vi "ParseXML.vi"(8 "error in (no error)":errorcluster, 11 "Node":string="<Sequential ID=\"1\">\n<Parallel ID=\"2\">\n<Wait ID=\"6\" Time=\"1.00\"/>\n<DriveForDistance Distance=\"4.00\" ID=\"3\" Speed=\"4.00\"/>\n</Parallel>\n<DrivePath ID=\"5\" Path=\"2C\"/>\n</Sequential>\n</Sequential>") -> (0 "error out":errorcluster)   [LabVIEW 2017]
uses:
  <vilib>/regexp/Match Regular Expression.xnode
panel:
  out "Node Name":string
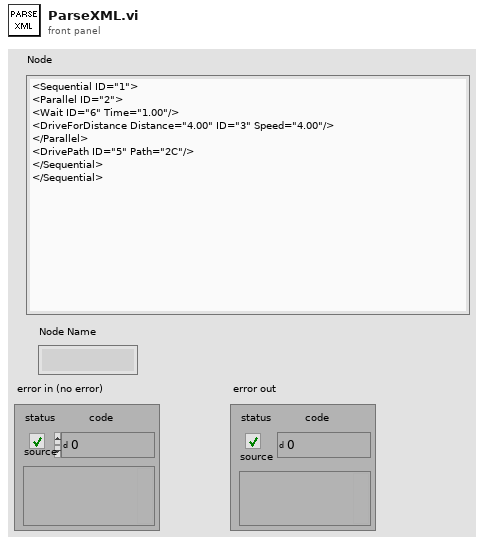
[diagram p1: front panel]
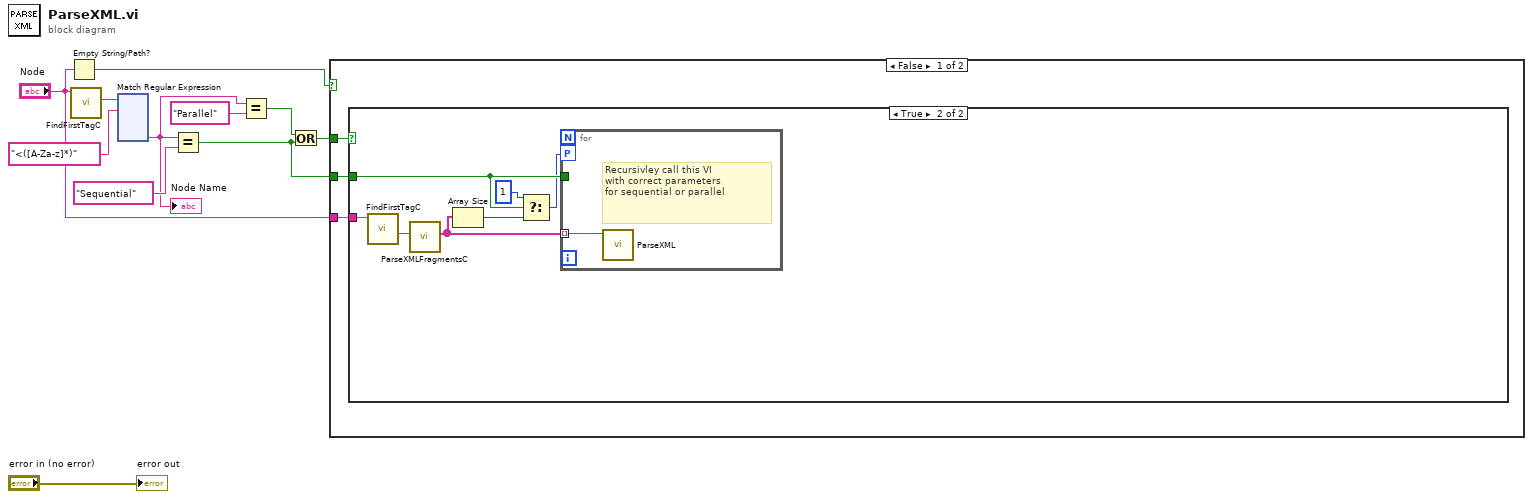
[diagram p0: block diagram]
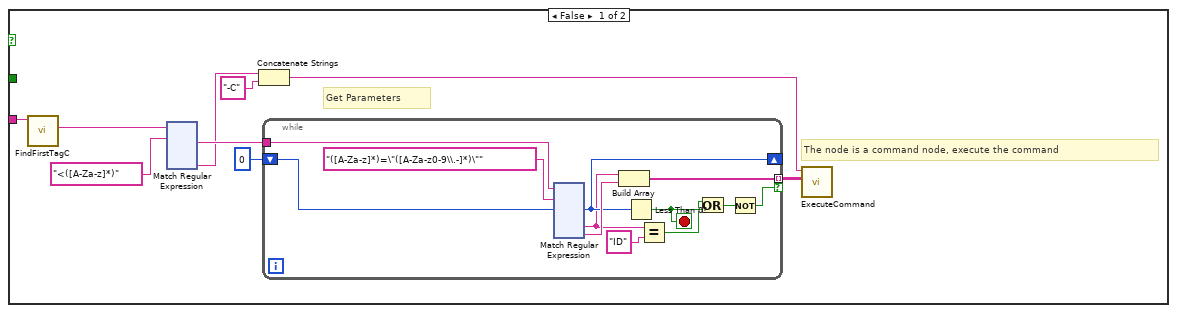
[diagram p2: hidden frame]
diagram:
  n1 = Empty String/Path?(string/path="Node") -> (empty?=w5:bool)
  n2 = call "FindFirstTagC.vi"("XML String In"="Node") -> ("tag"=w4:string)  [unwired: 1 in, 9 out]
  n3 = xnode "Match Regular Expression"("input string"=w4, "regular expression"="<([A-Za-z]*)") -> ("submatch 1"=w2:string)  [unwired: 4 in, 5 out]
  "Node Name" <- w2
  n4 = Equal?(x=w2, y="Sequential") -> (x = y?=w7:bool)
  n5 = Equal?(x=w2, y="Parallel") -> (x = y?=w9:bool)
  n6 = Or(x=w9, y=w7) -> (x .or. y?=w8:bool)
  n7 = case shown="False" w5 {
    tunnel: w8 -> [w14 _]
    tunnel: w7 -> [w13 _]
    tunnel: "Node" -> [w12 _]
    frame False {
      n8 = case shown="True" w14 {
        tunnel: w13 -> [_ w275]
        tunnel: w12 -> [w19 w270]
        frame False {
          # "Get Parameters"
          # "The node is a command node, execute the command"
          n9 = call "FindFirstTagC.vi"("XML String In"=w19) -> ("tag"=w22:string)  [unwired: 1 in, 9 out]
          n10 = xnode "Match Regular Expression"("input string"=w22, "regular expression"="<([A-Za-z]*)") -> ("after match"=w21:string, "submatch 1"=w18:string)  [unwired: 4 in, 4 out]
          n11 = Concatenate Strings(w18, "-C" ("string")) -> (w16:string)
          n12 = while {
            tunnel: w21 -> [w35]
            tunnel: [w31] -> w15 mode=indexing if=w29
            shift-right: [w30] -> _
            shift-left: 0 ("offset (0)") -> [w34]
            stop <- w27 stop-if-true
            n13 = xnode "Match Regular Expression"("input string"=w35, "regular expression"="([A-Za-z]*)=\"([A-Za-z0-9\\.-]*)\"", "offset (0)"=w34) -> ("offset past match"=w30:i32, "submatch 1"=w24:string, "submatch 2"=w32:string)  [unwired: 3 in, 4 out]
            n14 = Build Array(w24, w32) -> (w31:string[])
            n15 = Less Than 0?(x=w30) -> (x < 0?=w27:bool)
            n16 = Equal?(x=w24, y="ID") -> (x = y?=w25:bool)
            n17 = Or(x=w25, y=w27) -> (x .or. y?=w26:bool)
            n18 = Not(x=w26) -> (.not. x?=w29:bool)
          }
          n19 = call "ExecuteCommand.vi"("Params"=w15, "Command"=w16) -> ()  [unwired: 10 in]
        }
        frame True {
          n20 = call "FindFirstTagC.vi"("XML String In"=w270) -> ("after tag"=w269:string)  [unwired: 1 in, 9 out]
          n21 = call "ParseXMLFragmentsC.vi"("XML in"=w269) -> ("XML Elements"=w271:string[])  [unwired: 9 in, 1 out]
          n22 = Array Size(array=w271) -> (size(s)=w273:i32)
          n23 = Select(t=1, s=w275, f=w273) -> (s? t:f=w272:i32)
          n24 = for {
            tunnel: w271 -> [w276] mode=indexing
            tunnel: w275 -> [_]
            workers-P: w272 -> [_]
            # "Recursivley call this VI\nwith correct parameters\nfor sequential or parallel"
            n25 = call "ParseXML.vi"("Node"=w276) -> ()  [unwired: 10 in, 1 out]
          }
        }
      }
    }
    frame True {
    }
  }
  "error out" <- "error in (no error)"
